vi "Get_Process_Details.vi"(0 "Wash_Type":string, 5 "Process_Data":string[][](array[string])) -> (4 "Process":string[](array[string]), 6 "Time":dbl[](array[numeric]))   [LabVIEW 2023]
doc: "Used to get the washing details from the washing data and wash type"
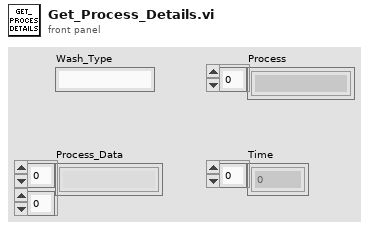
[diagram p1: front panel]
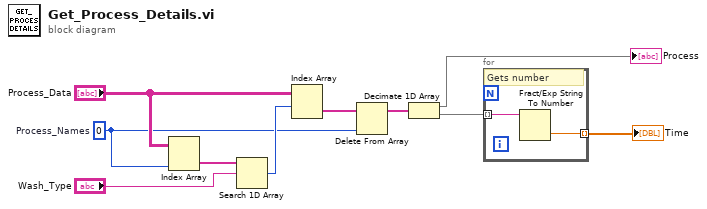
[diagram p0: block diagram]
diagram:
  w1 = 0  # Process_Names
  n1 = Index Array(array="Process_Data", index (col)=w1) -> (element=w2:string[])  [unwired: 1 in]
  n2 = Search 1D Array(1D array=w2, element="Wash_Type") -> (index of element=w4:i32)  [unwired: 1 in]
  n3 = Index Array(array="Process_Data", index (row)=w4) -> (element=w6:string[])  [unwired: 1 in]
  n4 = Delete From Array(array=w6, index=w1) -> (array with subset deleted=w7:string[])  [unwired: 1 in, 1 out]
  n5 = Decimate 1D Array(w7) -> (→"Process":string[], w8:string[])
  n6 = for {
    tunnel: w8 -> [w12] mode=indexing
    tunnel: [w11] -> w10 mode=indexing
    # "Gets number"
    n7 = Fract/Exp String To Number(string=w12) -> (number=w11:dbl)  [unwired: 3 in, 1 out]
  }
  "Time" <- w10
